vi "Init.vi"(8 "error in (no error)":errorcluster, 9 "SA Pin":string, 10 "Measurement Name":string) -> (0 "error out":errorcluster, 3 "TDSCDMA_ACP out":refnum<class "TDSCDMA_ACP.lvclass">)   [LabVIEW 2016, in "SeqAuto Evaluations.lvlib" / "TDSCDMA_ACP.lvclass"]
uses:
  TDSCDMA_ACP.lvclass
  C:/Sequence Automation/Plugins/SeqAuto IEvaluation.lvlibp/SeqAuto IEvaluation.lvclass
  TDSCDMA_ACP.lvclass/TDSCDMA_ACP.ctl
  Plugins/SeqAuto IEvaluation.lvlibp/Write Measurement Name.vi
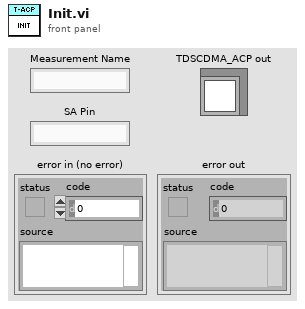
[diagram p1: front panel]
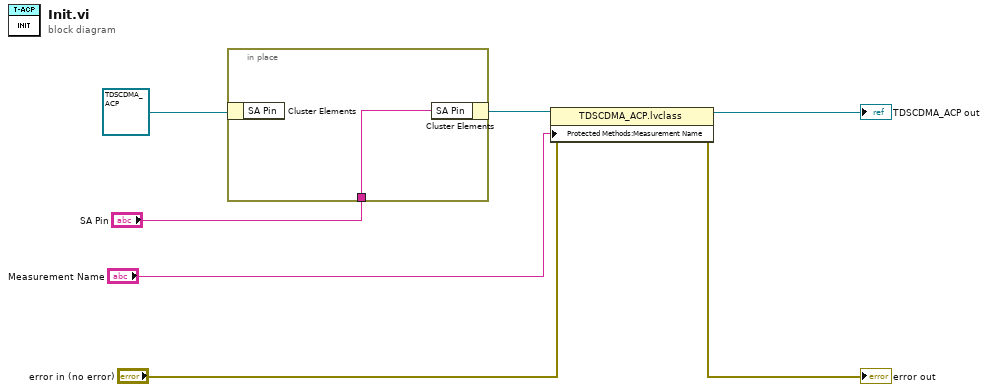
[diagram p0: block diagram]
diagram:
  n1 = in-place {
    in-place-border: "SA Pin" -> [w8]
    n2 = in-place-cluster #1(refnum<class "TDSCDMA_ACP.lvclass"> refnum ("TDSCDMA_ACP in")) -> ()  [unwired: 1 out]
    n3 = in-place-cluster #1("SA Pin"=w8) -> (w3:refnum<class "TDSCDMA_ACP.lvclass">)
  }
  n4 = property class="TDSCDMA_ACP.lvclass"(reference=w3, error in="error in (no error)", "Protected Methods:Measurement Name"="Measurement Name") -> (reference out=→"TDSCDMA_ACP out":refnum<class "TDSCDMA_ACP.lvclass">, error out=→"error out":errorcluster)
